vi "Halvorsen_HDiagram_New.vi"(11 "Initial Conditions":ext[](array[numeric])=[0.1, 0.1, 0.1]) -> ()   [LabVIEW 2016]
panel:
  in  "Method":i32=2
  out "Current h":ext=0.9999999999999999994
  in  "Inc h, с":ext=0.01
  in  "Parameters":ext[](array[numeric])=[0.1, 0.1, 0.1]
  in  "Tab Control":enum32{"Mode Analysis", "Time Domain"}(tab)
  out "Mode Analysis":cluster{ext[], dbl[]}[](graph)=[{[0.01, 0.02, 0.03, 0.04, 0.049999999999999999997, 0.059999999999999999995, 0.069999999999999999993, 0.07999999999999999999, 0.08999999999999999999, 0.09999999999999999999, 0.109999999999999999986, 0.119999999999999999984, 0.12999999999999999998, 0.13999999999999999999, 0.14999999999999999999, 0.16, 0.17, 0.18000000000000000001, 0.19000000000000000001, 0.20000000000000000002, 0.21000000000000000002, 0.22000000000000000003, 0.23000000000000000003, 0.24000000000000000004, 0.25000000000000000003, 0.26000000000000000002, 0.27000000000000000001, 0.28, 0.29, 0.29999999999999999998, 0.30999999999999999998, 0.31999999999999999997, 0.32999999999999999996, 0.33999999999999999995, 0.34999999999999999994, 0.35999999999999999993, 0.36999999999999999992, 0.37999999999999999991, 0.3899999999999999999, 0.3999999999999999999, 0.40999999999999999989, 0.41999999999999999988, 0.42999999999999999987, 0.43999999999999999986, 0.44999999999999999985, 0.45999999999999999984, 0.46999999999999999984, 0.47999999999999999983, 0.48999999999999999982, 0.4999999999999999998, 0.50999999999999999983, 0.51999999999999999982, 0.5299999999999999998, 0.5399999999999999998, 0.5499999999999999998, 0.5599999999999999998, 0.56999999999999999978, 0.57999999999999999977, 0.58999999999999999976, 0.59999999999999999975, 0.60999999999999999974, 0.61999999999999999973, 0.62999999999999999972, 0.6399999999999999997, 0.6499999999999999997, 0.6599999999999999997, 0.6699999999999999997, 0.67999999999999999968, 0.68999999999999999967, 0.69999999999999999966, 0.70999999999999999966, 0.71999999999999999965, 0.72999999999999999964, 0.73999999999999999963, 0.74999999999999999962, 0.7599999999999999996, 0.7699999999999999996, 0.7799999999999999996, 0.7899999999999999996, 0.79999999999999999958, 0.80999999999999999957, 0.81999999999999999956, 0.82999999999999999955, 0.83999999999999999954, 0.84999999999999999953, 0.85999999999999999953, 0.8699999999999999995, 0.8799999999999999995, 0.8899999999999999995, 0.8999999999999999995, 0.9099999999999999995, 0.91999999999999999947, 0.92999999999999999946, 0.93999999999999999946, 0.94999999999999999945, 0.95999999999999999944, 0.96999999999999999943, 0.9799999999999999994, 0.9899999999999999994], [22.0, 19.0, 21.0, 20.0, 19.0, 20.0, 21.0, 22.0, 21.0, 19.0, 19.0, 23.0, 18.0, 17.0, 23.0, 19.0, 23.0, 22.0, 18.0, 17.0, 18.0, 21.0, 20.0, 23.0, 19.0, 24.0, 17.0, 25.0, 22.0, 28.0, 21.0, 21.0, 22.0, 21.0, 19.0, 21.0, 24.0, 23.0, 19.0, 25.0, 26.0, 21.0, 23.0, 18.0, 25.0, 19.0, 22.0, 24.0, 20.0, 22.0, 27.0, 20.0, 25.0, 22.0, 21.0, 23.0, 26.0, 24.0, 27.0, 22.0, 23.0, 26.0, 23.0, 23.0, 24.0, 21.0, 21.0, 24.0, 23.0, 22.0, 24.0, 23.0, 22.0, 17.0, 22.0, 22.0, 19.0, 27.0, 23.0, 25.0, 20.0, 22.0, 21.0, 25.0, 22.0, 22.0, 21.0, 14.0, 17.0, 24.0, 27.0, 24.0, 21.0, 25.0, 22.0, 27.0, 20.0, 20.0, 22.0]}, {[0.01, 0.02, 0.03, 0.04, 0.049999999999999999997, 0.059999999999999999995, 0.069999999999999999993, 0.07999999999999999999, 0.08999999999999999999, 0.09999999999999999999, 0.109999999999999999986, 0.119999999999999999984, 0.12999999999999999998, 0.13999999999999999999, 0.14999999999999999999, 0.16, 0.17, 0.18000000000000000001, 0.19000000000000000001, 0.20000000000000000002, 0.21000000000000000002, 0.22000000000000000003, 0.23000000000000000003, 0.24000000000000000004, 0.25000000000000000003, 0.26000000000000000002, 0.27000000000000000001, 0.28, 0.29, 0.29999999999999999998, 0.30999999999999999998, 0.31999999999999999997, 0.32999999999999999996, 0.33999999999999999995, 0.34999999999999999994, 0.35999999999999999993, 0.36999999999999999992, 0.37999999999999999991, 0.3899999999999999999, 0.3999999999999999999, 0.40999999999999999989, 0.41999999999999999988, 0.42999999999999999987, 0.43999999999999999986, 0.44999999999999999985, 0.45999999999999999984, 0.46999999999999999984, 0.47999999999999999983, 0.48999999999999999982, 0.4999999999999999998, 0.50999999999999999983, 0.51999999999999999982, 0.5299999999999999998, 0.5399999999999999998, 0.5499999999999999998, 0.5599999999999999998, 0.56999999999999999978, 0.57999999999999999977, 0.58999999999999999976, 0.59999999999999999975, 0.60999999999999999974, 0.61999999999999999973, 0.62999999999999999972, 0.6399999999999999997, 0.6499999999999999997, 0.6599999999999999997, 0.6699999999999999997, 0.67999999999999999968, 0.68999999999999999967, 0.69999999999999999966, 0.70999999999999999966, 0.71999999999999999965, 0.72999999999999999964, 0.73999999999999999963, 0.74999999999999999962, 0.7599999999999999996, 0.7699999999999999996, 0.7799999999999999996, 0.7899999999999999996, 0.79999999999999999958, 0.80999999999999999957, 0.81999999999999999956, 0.82999999999999999955, 0.83999999999999999954, 0.84999999999999999953, 0.85999999999999999953, 0.8699999999999999995, 0.8799999999999999995, 0.8899999999999999995, 0.8999999999999999995, 0.9099999999999999995, 0.91999999999999999947, 0.92999999999999999946, 0.93999999999999999946, 0.94999999999999999945, 0.95999999999999999944, 0.96999999999999999943, 0.9799999999999999994, 0.9899999999999999994], [23.0, 18.0, 21.0, 20.0, 19.0, 21.0, 20.0, 21.0, 21.0, 18.0, 18.0, 22.0, 19.0, 17.0, 23.0, 20.0, 22.0, 22.0, 19.0, 16.0, 19.0, 21.0, 20.0, 23.0, 20.0, 24.0, 17.0, 26.0, 21.0, 26.0, 22.0, 21.0, 22.0, 22.0, 17.0, 21.0, 24.0, 23.0, 19.0, 22.0, 24.0, 21.0, 23.0, 17.0, 24.0, 20.0, 22.0, 25.0, 20.0, 18.0, 25.0, 19.0, 25.0, 21.0, 22.0, 23.0, 27.0, 25.0, 27.0, 19.0, 22.0, 26.0, 22.0, 24.0, 24.0, 18.0, 21.0, 25.0, 24.0, 21.0, 25.0, 24.0, 23.0, 16.0, 20.0, 22.0, 19.0, 23.0, 22.0, 24.0, 20.0, 21.0, 19.0, 25.0, 19.0, 21.0, 21.0, 14.0, 18.0, 21.0, 24.0, 23.0, 21.0, 24.0, 22.0, 27.0, 19.0, 20.0, 20.0]}]
  out "Waveform Graph":ext[][](graph)
  out "Bifurcation Diagram":cluster{ext[], ext[]}(graph)
  in  "Final h":dbl=1.0
  in  "Variable":u16(ring) items=["x", "y", "z"]
  in  "Время, с":ext=500.0
  in  "tolerance":ext=1e-11
  in  "Шаг h, с":ext=0.01
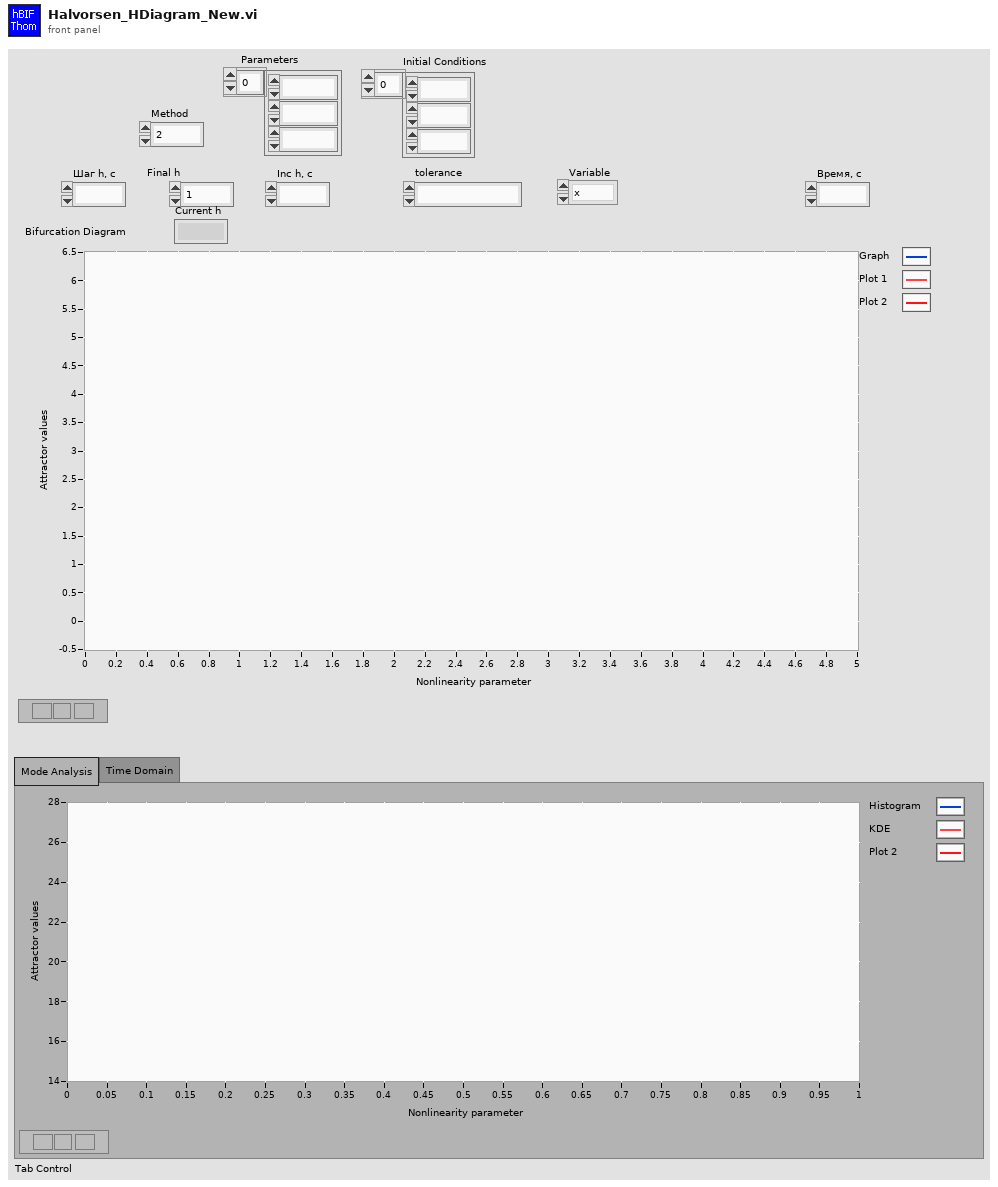
[diagram p1: front panel]
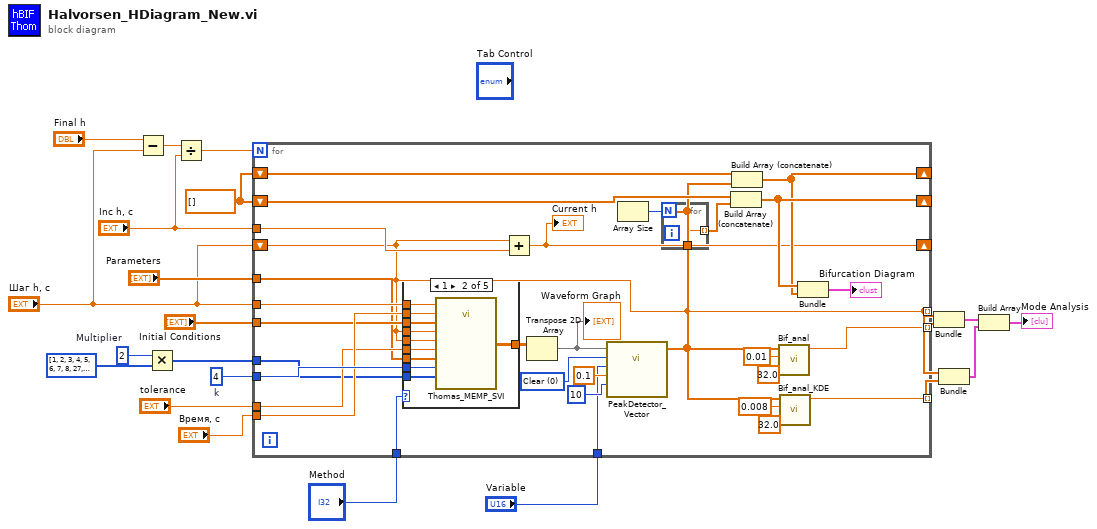
[diagram p0: block diagram]
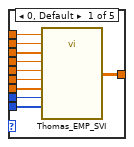
[diagram p2: hidden frame]
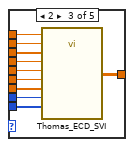
[diagram p3: hidden frame]
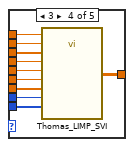
[diagram p4: hidden frame]
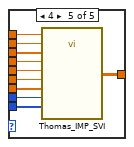
[diagram p5: hidden frame]
diagram:
  w14 = ext[] []
  w15 = 4  # k
  w18 = 2  # Multiplier
  n1 = Subtract(x="Final h", y="Шаг h, с") -> (x-y=w5:ext)
  n2 = Multiply(x=w18, y=i32[] [1, 2, 3, 4, 5, 6, 7, 8, 27, 30, 33] ("n")) -> (x*y=w16:i32[])
  n3 = Divide(x=w5, y="Inc h, с") -> (x/y=w3:ext)
  n4 = for {
    N: w3 -> [_]
    tunnel: w15 -> [w53]
    tunnel: "Шаг h, с" -> [w44]
    tunnel: "Время, с" -> [w52]
    tunnel: "tolerance" -> [w51]
    tunnel: w16 -> [w50]
    tunnel: "Initial Conditions" -> [w49]
    shift-right: [w24] -> _
    shift-left: "Шаг h, с" -> [w25]
    tunnel: [w43] -> w13 mode=indexing
    tunnel: "Variable" -> [w42]
    shift-right: [w35] -> _
    shift-left: w14 -> [w40]
    shift-right: [w36] -> _
    shift-left: w14 -> [w39]
    tunnel: [w25] -> w10 mode=indexing
    tunnel: [w29] -> w9 mode=indexing
    tunnel: "Parameters" -> [w27]
    tunnel: "Inc h, с" -> [w26]
    tunnel: "Method" -> [w23]
    w47 = u16 0 items=["Clear", "Absolute", "Positive"] ("Signal Mode")
    n5 = case shown="1" w23 {
      tunnel: w53 -> [w64 w74 w84 w94 w104]
      tunnel: w52 -> [w63 w73 w83 w93 w103]
      tunnel: w51 -> [w62 w72 w82 w92 w102]
      tunnel: w25 -> [w61 w71 w81 w91 w101]
      tunnel: w25 -> [w60 w70 w80 w90 w100]
      tunnel: w50 -> [w59 w69 w79 w89 w99]
      tunnel: w49 -> [w58 w68 w78 w88 w98]
      tunnel: [w57 w67 w77 w87 w97] -> w48
      tunnel: w44 -> [w56 w66 w76 w86 w96]
      tunnel: w27 -> [w55 w65 w75 w85 w95]
      frame 0, Default {
        n6 = call "Thomas_EMP_SVI.vi"("Шаг h, с"=w56, "n"=w59, "k"=w64, "Parameter_Vector"=w55, "Время, с"=w63, "Initial Conditions"=w58, "Hmin"=w61, "Hmax"=w60, "tolerance"=w62) -> ("Solution"=w57:ext[][])  [unwired: 6 in]
      }
      frame 1 {
        n7 = call "Thomas_MEMP_SVI.vi"("Шаг h, с"=w66, "n"=w69, "k"=w74, "Parameter_Vector"=w65, "Время, с"=w73, "Initial Conditions"=w68, "Hmin"=w71, "Hmax"=w70, "tolerance"=w72) -> ("Solution"=w67:ext[][])  [unwired: 6 in]
      }
      frame 2 {
        n8 = call "Thomas_ECD_SVI.vi"("Шаг h, с"=w76, "n"=w79, "k"=w84, "Parameter_Vector"=w75, "Время, с"=w83, "Initial Conditions"=w78, "Hmin"=w81, "Hmax"=w80, "tolerance"=w82) -> ("Solution"=w77:ext[][])  [unwired: 6 in]
      }
      frame 3 {
        n9 = call "Thomas_LIMP_SVI.vi"("Шаг h, с"=w86, "n"=w89, "k"=w94, "Parameter_Vector"=w85, "Время, с"=w93, "Initial Conditions"=w88, "Hmin"=w91, "Hmax"=w90, "tolerance"=w92) -> ("Solution"=w87:ext[][])  [unwired: 6 in]
      }
      frame 4 {
        n10 = call "Thomas_IMP_SVI.vi"("Шаг h, с"=w96, "n"=w99, "k"=w104, "Parameter_Vector"=w95, "Время, с"=w103, "Initial Conditions"=w98, "Hmin"=w101, "Hmax"=w100, "tolerance"=w102) -> ("Solution"=w97:ext[][])  [unwired: 6 in]
      }
    }
    n11 = Add(x=w25, y=w26) -> (x+y=w24:ext)
    "Current h" <- w24
    n12 = Transpose 2D Array(2D array=w48) -> (transposed array=w28:ext[][])
    "Waveform Graph" <- w28
    n13 = call "PeakDetector_Vector.vi"("threshold"=0.1, "FWD cut length"=10, "Variable_Num"=w42, "Signal Mode"=w47, "Input signal"=w28) -> ("Out signal"=w30:dbl[])  [unwired: 5 in, 1 out]
    n14 = Array Size(array=w30) -> (size(s)=w41:i32)
    n15 = for {
      N: w41 -> [_]
      tunnel: [w54] -> w37 mode=indexing
      tunnel: w25 -> [w54]
    }
    n16 = Build Array (concatenate)(w39, w37) -> (w36:ext[])
    n17 = Build Array (concatenate)(w40, w30) -> (w35:ext[])
    n18 = call "Bif_anal.vi"("n"=32.0, "Treshold"=0.01, "X"=w30) -> ("Y"=w43:dbl)  [unwired: 7 in, 1 out]
    n19 = call "Bif_anal_KDE.vi"("n"=32.0, "Manual h"=0.008 ("Treshold"), "X"=w30) -> ("Y"=w29:dbl)  [unwired: 7 in, 1 out]
    n20 = Bundle(w36, w35) -> (→"Bifurcation Diagram":cluster{ext[], ext[]})  [unwired: 1 in]
  }
  n21 = Bundle(w10, w13) -> (w12:cluster{ext[], dbl[]})  [unwired: 1 in]
  n22 = Bundle(w10, w9) -> (w8:cluster{ext[], dbl[]})  [unwired: 1 in]
  n23 = Build Array(w12, w8) -> (→"Mode Analysis":cluster{ext[], dbl[]}[])
